vi "test - add key in sperated but same name session.vi"(8 "error in (no error)":errorcluster, 11 "TestCase in":refnum<class "labview-config-library.lvclass">) -> (0 "error out":errorcluster, 3 "TestCase out":refnum<class "labview-config-library.lvclass">)   [LabVIEW 2017, in "labview-config-library.lvclass"]
uses:
  labview-config-library.lvclass
  <vilib>/addons/_JKI Toolkits/VI Tester/TestCase.llb/TestCase.lvclass
  INI-Static-Variable-Support/LabVIEW-Config/LabVIEW-Config.lvclass
  <userlib>/_NEVSTOP/Communicable State Machine(CSM)/Communicable State Machine.lvlib
  INI-Static-Variable-Support/LabVIEW-Config/Write Key (Raw).vi
  C:/Program Files (x86)/National Instruments/LabVIEW 2017/vi.lib/addons/_JKI Toolkits/VI Tester/TestCase.llb/TestCase.lvclass
panel:
  in  "Tab Control":enum32{"Page 1", "Page 2", "Page 3"}(tab)
  out "text":string
  out "Key Names":string[](array[string])
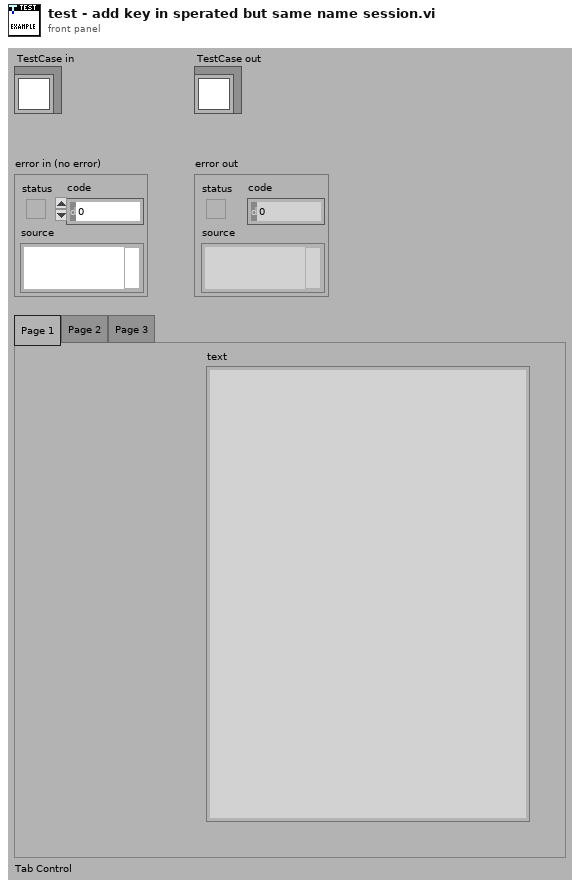
[diagram p1: front panel]
types:
  T1 = typedef "LabVIEW-Config.lvlib/LabVIEW-Config.lvclass/Config.ctl" = cluster{"Path":path, "Lines":string[], "Tokens":T2[], "Modified?":bool, "Cache":cluster{"Valid?":bool, "Key Information":T3[]}}
  T2 = typedef "LabVIEW-Config.lvlib/LabVIEW-Config.lvclass/LineToken.ctl" = enum8{"comment", "section", "key", "more"}
  T3 = typedef "LabVIEW-Config.lvlib/LabVIEW-Config.lvclass/KeyInfo.ctl" = cluster{"Key Indexes":cluster{"Indexes":i32[]}[], "Session Found?":bool, "Key found?":bool, "Session Index":i32}
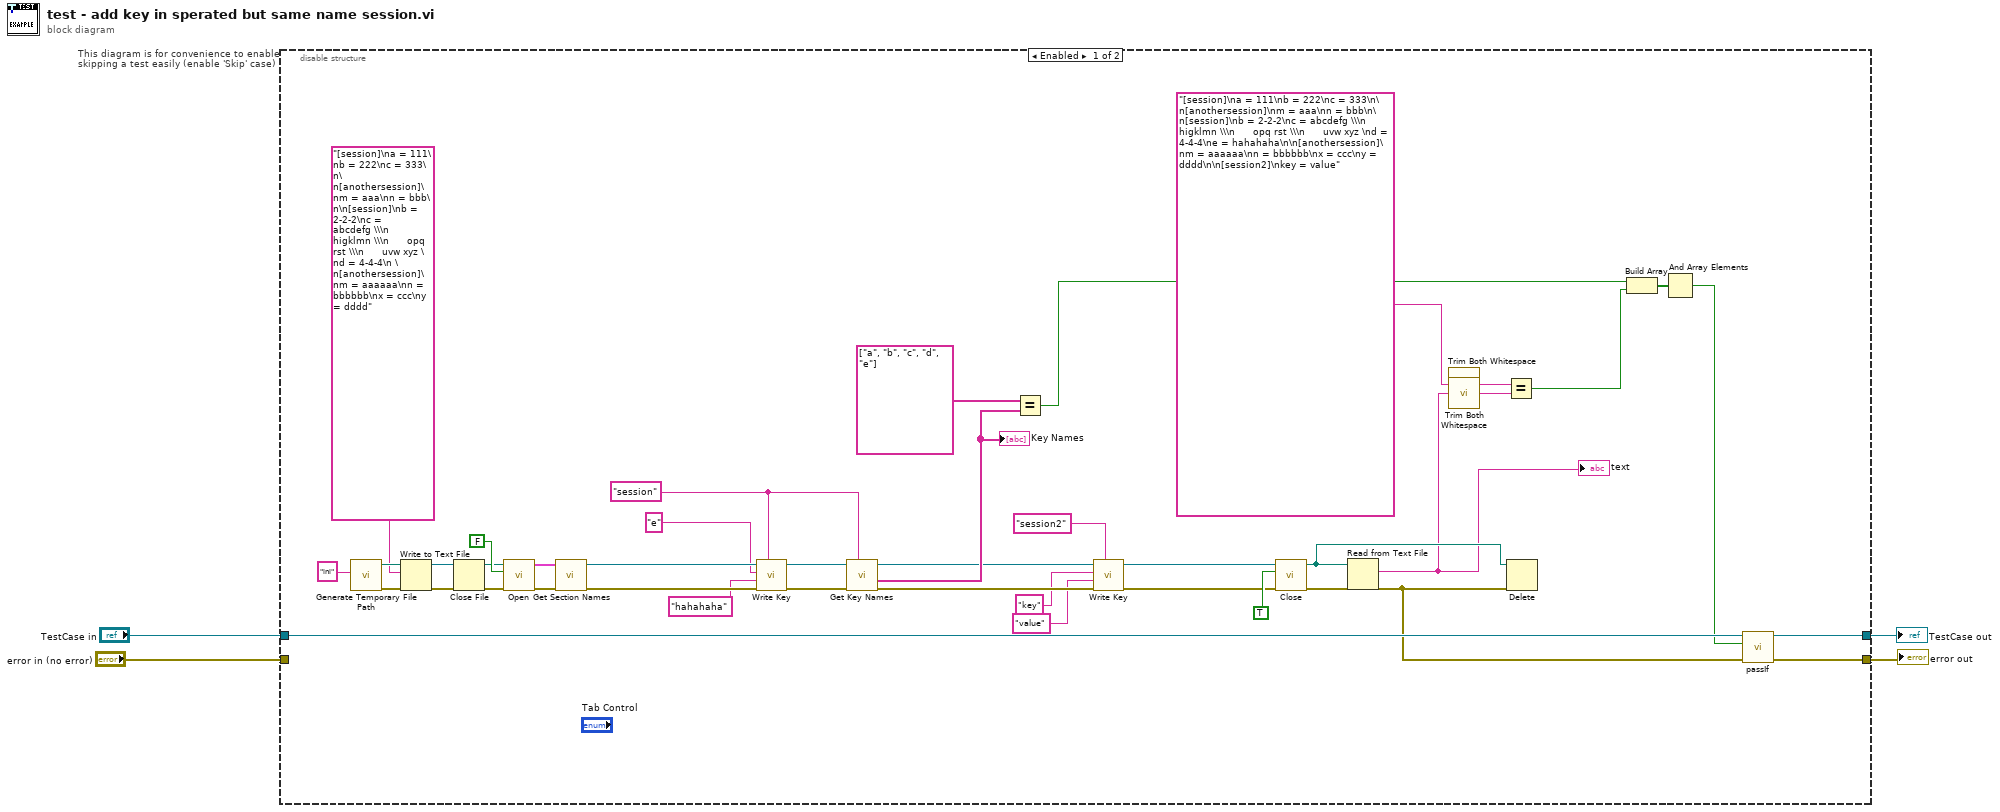
[diagram p0: block diagram]
diagram:
  n1 = disable-structure "This diagram is for convenience to enable skipping a test easily (enable 'Skip' case)" shown="Enabled" {
    disable-tunnel: "TestCase in" -> [w46 w50]
    disable-tunnel: [w45 w48] -> w1
    disable-tunnel: [w44 w49] -> w3
    disable-tunnel: "error in (no error)" -> [_ w47]
    frame Enabled {
      w19 = "session" ("Section Name")
      # "Create temporary ini file"
      n2 = call <vilib>:"Generate Temporary File Path.vi"("Temporary File Extension (tmp)"="ini") -> ("error out"=w41:errorcluster, "Unique Temporary File Path"=w38:path)  [unwired: 9 in]
      n3 = Write to Text File(file (use dialog)=w38, text="[session]\na = 111\nb = 222\nc = 333\n\n[anothersession]\nm = aaa\nn = bbb\n\n[session]\nb = 2-2-2\nc = abcdefg \\\n      higklmn \\\n      opq rst \\\n      uvw xyz \nd = 4-4-4\n \n[anothersession]\nm = aaaaaa\nn = bbbbbb\nx = ccc\ny = dddd", error in=w41) -> (refnum out=w37:refnum<file>, error out=w39:errorcluster)  [unwired: 1 in, 1 out]
      n4 = Close File(refnum=w37, error in=w39) -> (path=w34:path, error out=w35:errorcluster)
      n5 = call "Open.vi"("error in (no error)"=w35, "Create if not exists? (T)"=FALSE, "Path"=w34) -> ("error out"=w32:errorcluster, "Config"=w33:T1)  [unwired: 5 in, 2 out]
      n6 = call "Get Section Names.vi"("error in (no error)"=w32, "Config in"=w33) -> ("error out"=w21:errorcluster, "Config out"=w31:refnum<class "LabVIEW-Config.lvclass">)  [unwired: 7 in, 1 out]
      n7 = call-poly "Write Key.vi"("Section Name"=w19, "error in (no error)"=w21, "Content"="hahahaha" ("Value"), "Key Name"="e", "Config in"=w31) -> ("error out"=w20:errorcluster, "Config out"=w22:refnum<class "LabVIEW-Config.lvclass">)  [unwired: 4 in, 1 out]
      n8 = call "Get Key Names.vi"("Section Name"=w19, "error in (no error)"=w20, "Config in"=w22) -> ("error out"=w10:errorcluster, "Key Names"=w27:string[], "Config out"=w11:refnum<class "LabVIEW-Config.lvclass">)  [unwired: 5 in, 1 out]
      "Key Names" <- w27
      n9 = Equal?(x=string[] ["a", "b", "c", "d", "e"] ("Key Names"), y=w27) -> (x = y?=w26:bool)
      n10 = call-poly "Write Key.vi"("Section Name"="session2", "error in (no error)"=w10, "Content"="value", "Key Name"="key", "Config in"=w11) -> ("error out"=w9:errorcluster, "Config out"=w8:refnum<class "LabVIEW-Config.lvclass">)  [unwired: 4 in, 1 out]
      n11 = call "Close.vi"("error in (no error)"=w9, "Write if modified? (T)"=TRUE, "Config"=w8) -> ("error out"=w24:errorcluster, "Path"=w25:path)  [unwired: 7 in]
      n12 = Read from Text File(file (use dialog)=w25, error in=w24) -> (text=w16:string, error out=w23:errorcluster)  [unwired: 2 in, 2 out]
      "text" <- w16
      n13 = call <userlib>:"Trim Both Whitespace.vi"("string"="[session]\na = 111\nb = 222\nc = 333\n\n[anothersession]\nm = aaa\nn = bbb\n\n[session]\nb = 2-2-2\nc = abcdefg \\\n      higklmn \\\n      opq rst \\\n      uvw xyz \nd = 4-4-4\ne = hahahaha\n\n[anothersession]\nm = aaaaaa\nn = bbbbbb\nx = ccc\ny = dddd\n\n[session2]\nkey = value") -> ("trimmed string"=w12:string)  [unwired: 1 in]
      n14 = call <userlib>:"Trim Both Whitespace.vi"("string"=w16) -> ("trimmed string"=w13:string)  [unwired: 1 in]
      n15 = Equal?(x=w12, y=w13) -> (x = y?=w15:bool)
      n16 = Delete(path (use dialog)=w25, error in=w23) -> ()  [unwired: 3 in, 3 out]
      n17 = Build Array(w26, w15) -> (w30:bool[])
      n18 = And Array Elements(Boolean array=w30) -> (logical AND=w29:bool)
      n19 = call-dynamic "passIf.vi"("error in (no error)"=w23, "pass"=w29, "TestCase in"=w46) -> ("error out"=w44:errorcluster, "TestCase out"=w45:refnum<class "labview-config-library.lvclass">)  [unwired: 7 in]
    }
    frame Disabled {
      # "skip test result while test is under development"
      n20 = call <vilib>:"skip.vi"("error in (no error)"=w47, "TestCase in"=w50) -> ("error out"=w49:errorcluster, "TestCase out"=w48:refnum<class "labview-config-library.lvclass">)  [unwired: 8 in]
    }
  }
  "error out" <- w3
  "TestCase out" <- w1
